vi "acquireData_1chan.vi"() -> ()   [LabVIEW 2023]
uses:
  <vilib>/DAQmx/read.llb/DAQmx Read (Analog Wfm 1Chan NSamp).vi
  <vilib>/DAQmx/create/channels.llb/DAQmx Create Channel (AI-Voltage-Basic).vi
  <vilib>/DAQmx/configure/timing.llb/DAQmx Timing (Sample Clock).vi
  <vilib>/DAQmx/miscellaneous.llb/DAQmx Fill In Error Info.vi
  <resource>/objmgr/daqmx.rc
panel:
  out "Waveform Graph":waveform(dbl)(graph)
  in  "Play Measured Signal?":bool
  in  "AI Channel Name":string="/ai1"
  out "data":waveform(dbl)
  out "error out":errorcluster
  in  "Sampling Rate":dbl
  in  "Receive Duration":dbl
  in  "DAQmx Device Name":tag
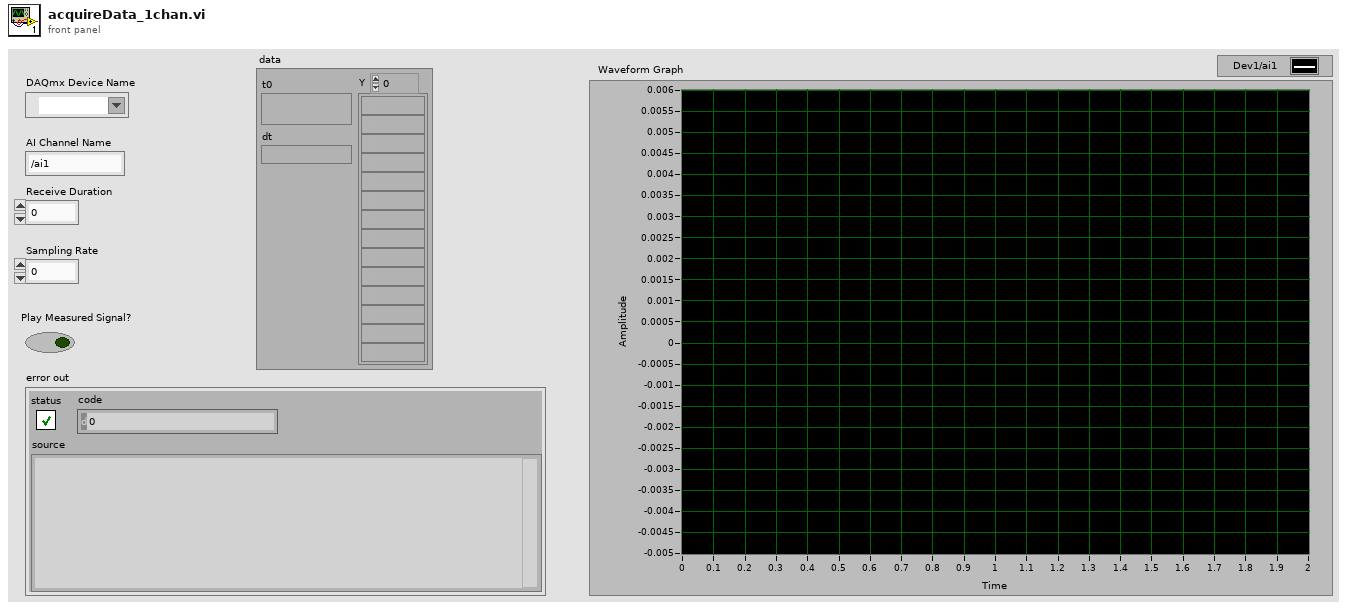
[diagram p1: front panel]
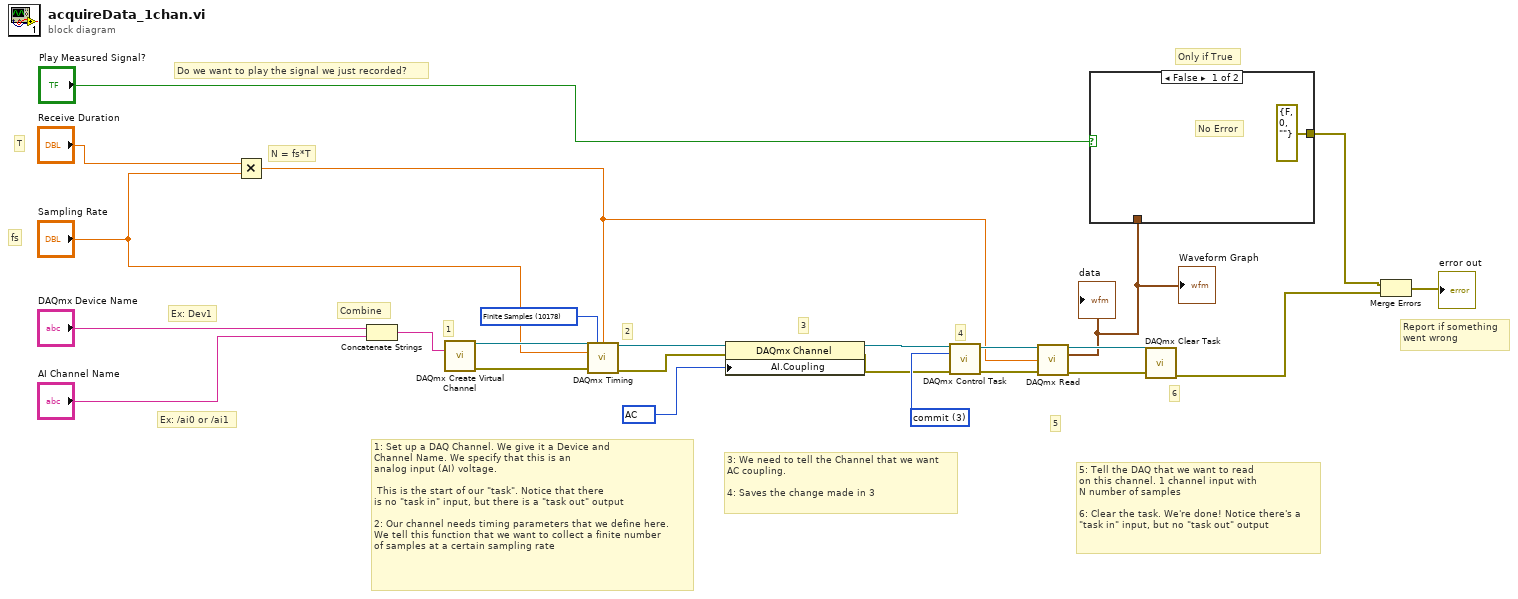
[diagram p0: block diagram]
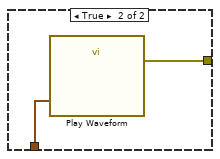
[diagram p2: hidden frame]
diagram:
  w18 = 10045 items=["AC"=10045, "DC"=10050, "GND"=10066] ("AI.Coupling")
  w19 = 10178 items=["Finite Samples"=10178, "Continuous Samples"=10123, "Hardware Timed Single Point"=12522] ("sample mode")
  w21 = 3 items=["verify"=2, "reserve"=4, "commit"=3, "unreserve"=5, "abort"=6] ("action")
  # "Only if True"
  # "5: Tell the DAQ that we want to read\non this channel. 1 channel input with\nN number of samples\n\n6: Clear the task. We're done! Notice there's a \n\"task in\" input, but no \"task out\" output"
  # "Report if something\nwent wrong"
  # "Do we want to play the signal we just recorded?"
  # "6"
  # "5"
  # "3: We need to tell the Channel that we want\nAC coupling.\n\n4: Saves the change made in 3"
  # "1: Set up a DAQ Channel. We give it a Device and \nChannel Name. We specify that this is an \nanalog input (AI) voltage.\n\n This is the start of our \"task\". Notice that there\nis no \"task in\" input, but there is a \"task out\" output\n\n2: Our channel needs timing parameters that we define here.\nWe tell this function that we want to collect a finite number\nof samples at a certain sampling rate"
  # "4"
  # "3"
  # "2"
  # "1"
  # "Ex: Dev1"
  # "Ex: /ai0 or /ai1"
  # "Combine"
  # "N = fs*T"
  # "T"
  # "fs"
  n1 = Multiply(x="Receive Duration", y="Sampling Rate") -> (x*y=w8:dbl)
  n2 = Concatenate Strings("DAQmx Device Name", "AI Channel Name") -> (w23:string)
  n3 = call-poly <vilib>:"DAQmx Create Virtual Channel.vi"("physical channels"=w23) -> ("task out"=w24:refnum<k21>, "error out"=w22:errorcluster)  [unwired: 13 in]
  n4 = call-poly <vilib>:"DAQmx Timing.vi"("task/channels in"=w24, "sample mode"=w19, "samples per channel"=w8, "rate"="Sampling Rate", "error in"=w22) -> ("task out"=w17:refnum<k21>, "error out"=w16:errorcluster)  [unwired: 9 in]
  n5 = property class="DAQmx Channel"(reference=w17, error in=w16, "AI.Coupling"=w18) -> (reference out=w15:refnum<k21>, error out=w14:errorcluster)
  n6 = call <vilib>:"DAQmx Control Task.vi"("task/channels in"=w15, "action"=w21, "error in"=w14) -> ("task out"=w13:refnum<k21>, "error out"=w12:errorcluster)  [unwired: 11 in]
  n7 = call-poly <vilib>:"DAQmx Read.vi"("task/channels in"=w13, "number of samples per channel"=w8, "error in"=w12) -> ("task out"=w11:refnum<k21>, "data"=w1:waveform(dbl), "error out"=w10:errorcluster)  [unwired: 10 in]
  "data" <- w1
  "Waveform Graph" <- w1
  n8 = case shown="False" "Play Measured Signal?" {
    tunnel: w1 -> [_ w27]
    tunnel: [errorcluster {"status"=FALSE, "code"=0, "source"=""} ("error out") w26] -> w3
    frame False {
      # "No Error"
    }
    frame True {
      n9 = call "Play Waveform"("Data"=w27) -> ("error out"=w26:errorcluster)  [unwired: 18 in]
    }
  }
  n10 = call <vilib>:"DAQmx Clear Task.vi"("task in"=w11, "error in"=w10) -> ("error out"=w4:errorcluster)  [unwired: 13 in]
  n11 = Merge Errors(w3, w4) -> (→"error out":errorcluster)
